vi "ALTS-2015 Decode User Password for version 2.vi"(10 "User Value":string, 11 "User Name":string) -> (3 "User Info":T1)   [LabVIEW 2013]
uses:
  Controls/ALTS-2015 User Info.ctl
  Controls/ALTS-2015 User Group Enum2.ctl
panel:
  # "Inputs"
  # "Outputs"
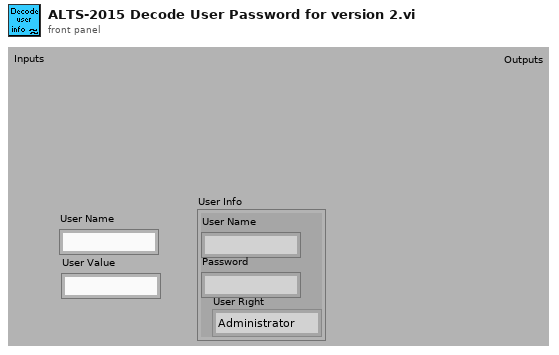
[diagram p1: front panel]
types:
  T1 = typedef "ALTS-2015 User Info.ctl" = cluster{"User Name":string, "Password":string, "User Right":T2}
  T2 = typedef "ALTS-2015 User Group Enum2.ctl" = enum16{"Administrator", "Super User", "Operator"}
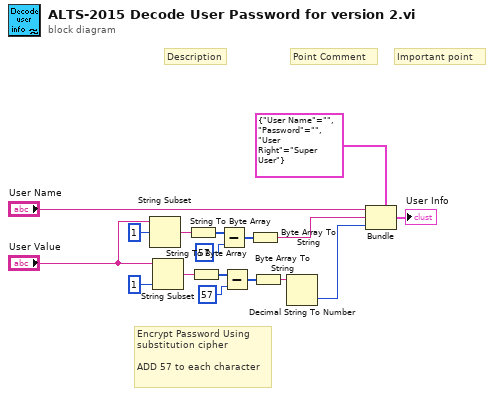
[diagram p0: block diagram]
diagram:
  # "Encrypt Password Using\nsubstitution cipher\n\nADD 57 to each character"
  # "Point Comment"
  # "Important point"
  # "Description"
  n1 = String Subset(string="User Value", offset (0)=1) -> (substring=w14:string)  [unwired: 1 in]
  n2 = String Subset(string="User Value", length (rest)=1 ("offset (0)")) -> (substring=w8:string)  [unwired: 1 in]
  n3 = String To Byte Array(string=w14) -> (unsigned byte array=w15:u8[])
  n4 = String To Byte Array(string=w8) -> (unsigned byte array=w11:u8[])
  n5 = Subtract(x=w15, y=57) -> (x-y=w17:i32[])
  n6 = Subtract(x=w11, y=57) -> (x-y=w9:i32[])
  n7 = Byte Array To String(unsigned byte array=w17) -> (string=w6:string)
  n8 = Byte Array To String(unsigned byte array=w9) -> (string=w7:string)
  n9 = Decimal String To Number(string=w7) -> (number=w5:i32)  [unwired: 2 in, 1 out]
  n10 = Bundle(cluster=T1 {"User Name"="", "Password"="", "User Right"=enum."Super User"} ("User"), "User Name"="User Name", "Password"=w6, "User Right"=w5) -> (→"User Info":T1)
